vi "channel_producer_dbl.vi"(4 "Enable":bool, 5 "Error In":errorcluster, 6 "Data":dbl[][](array[numeric]), 7 "Channels Names":string[](array[string]), 8 "Group Name":string) -> (0 "Error Out":errorcluster, 2 "TDMS Channel":T1)   [LabVIEW 2020]
uses:
  <extravilib>/ChannelInstances/Messenger-c(str,a[.](str),var)/))Channel.ctl
  <extravilib>/ChannelInstances/Messenger-c(str,a[.](str),var)/Write With Abort.vi
  <extravilib>/ChannelInstances/Messenger-c(str,a[.](str),var)/Endpoint.vi
  <extravilib>/ChannelInstances/Messenger-c(str,a[.](str),var).lvlib
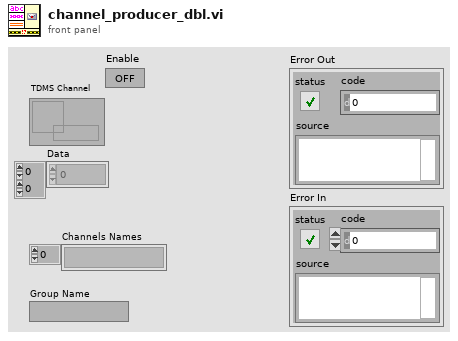
[diagram p1: front panel]
types:
  T1 = typedef "Messenger-c(str,a[.](str),var).lvlib/))Channel.ctl" = refnum<queue>
  T2 = cluster{"Group Name":string, "Channels Names":string[], "Variant":variant}
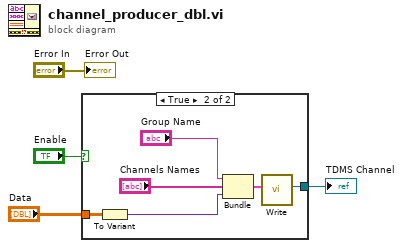
[diagram p0: block diagram]
diagram:
  n1 = case shown="True" "Enable" {
    tunnel: [_ w7] -> w4
    tunnel: "Data" -> [_ w6]
    frame False {
    }
    frame True {
      n2 = To Variant(anything=w6) -> (Variant=w5:variant)
      n3 = Bundle("Group Name"="Group Name", "Channels Names"="Channels Names", "Variant"=w5) -> (w8:T2)  [unwired: 1 in]
      n4 = call <extravilib>:"Write.vi"("element"=w8) -> ("channel"=w7:T1)  [unwired: 8 in, 2 out]
    }
  }
  "TDMS Channel" <- w4
  "Error Out" <- "Error In"
